vi "LiCor_poller.vi"(11 "LiCor session in":T1={"VISA resource out"="COM12", "error out"={"status"=FALSE, "code"=0, "source"=""}}) -> (0 "pCO2 out":dbl, 1 "data array":dbl[](array[numeric]), 2 "read string":string, 3 "LiCor session out":T1={"VISA resource out"="COM12", "error out"={"status"=FALSE, "code"=0, "source"=""}}, 4 "Integral out":dbl, 5 "actual bytes read":u32)   [LabVIEW 2010]
panel:
  # "LiCor Poller\n\nThis VI is a simple VI which completes a single poll of data from the LI-7000 LiCor instrument. It should follow a LiCor_init VI in whatever custom VI it is placed in - this will correctly initialize all the necessary values for successful operation. This VI spits out both raw data text as well as data in the form of an array."
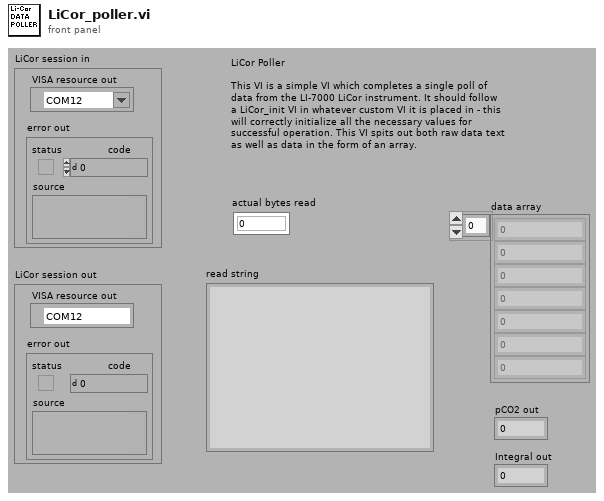
[diagram p1: front panel]
types:
  T1 = cluster{"VISA resource out":refnum<visa-resource-name>, "error out":errorcluster}
  T2 = cluster{"VISA session out":refnum<visa-resource-name>, "error out":errorcluster}
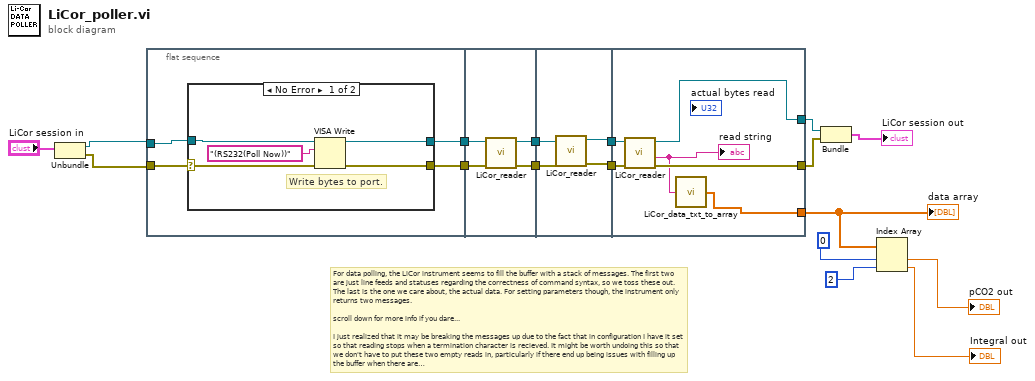
[diagram p0: block diagram]
diagram:
  # "For data polling, the LiCor instrument seems to fill the buffer with a stack of messages. The first two are just line feeds and statuses regarding the correctness of command syntax, so we toss these out. The last is the one we care about, the actual data. For setting parameters though, the instrument only returns two messages.\n\nscroll down for more info if you dare... \n\nI just realized that it may be breaking the messages up due to the fact that in configuration I have it set so that reading stops when a termination character is recieved. It might be worth undoing this so that we don't have to put these two empty reads in, particularly if there end up being issues with filling up the buffer when there are\n\nSorry for posting this as flow of thought, but if anyone is digging down this deep it may be useful. I just went into Advanced serial Write and Read and played around with some of the settings (ASRL End In, Supress End Enable, TermChar Enable and possible one or two others). Through some combination (which I think may have been accidental and I have not been able to reproduce though I haven't tried very hard - there may have been another setting I played with as well) I was able to get it to return both of the messages together (from a (Display(BackLt 1)) command), but I also got a timeout error from this. Trying to reset these values to ones that would make shut off the read termination, I was unable to reproduce the error, or get the read termination to end. Anyway, this isn't that important - I have things working. I just mention this in case someone has troubles down the road and needs to shoot them. It's also something of a matter of simple curiosity regarding what was causing the issues before. Nuff said..."
  n1 = Unbundle("LiCor session in") -> ("VISA resource out"=w10:refnum<visa-resource-name>, "error out"=w9:errorcluster)
  n2 = flat-sequence {
    tunnel: w10 -> [w21]
    tunnel: w9 -> [w20]
    tunnel: [w19] -> w17
    tunnel: [w18] -> w16
    tunnel: w17 -> [w32]
    tunnel: w16 -> [w31]
    tunnel: [w30] -> w15
    tunnel: [w29] -> w13
    tunnel: w15 -> [w36]
    tunnel: [w34] -> w14
    tunnel: w13 -> [w35]
    tunnel: [w33] -> w12
    tunnel: w14 -> [w42]
    tunnel: w12 -> [w41]
    tunnel: [w40] -> w8
    tunnel: [w39] -> w7
    tunnel: [w37] -> w3
    frame #0 {
      n3 = case shown="No Error" w20 {
        selector: w20 -> [w22 w28]
        tunnel: [w26 w27] -> w19
        tunnel: [w25 w28] -> w18
        tunnel: w21 -> [w23 w27]
        frame No Error {
          # "Write bytes to port."
          n4 = VISA Write(VISA resource name=w23, write buffer="(RS232(Poll Now))" ("string to write"), error in (no error)=w22) -> (VISA resource name out=w26:refnum<visa-resource-name>, error out=w25:errorcluster)  [unwired: 1 out]
        }
        frame Error {
        }
      }
    }
    frame #1 {
      n5 = call "LiCor_reader.vi"("error in"=w31, "VISA session in"=w32) -> ("error out"=w29:errorcluster, "VISA session out"=w30:refnum<visa-resource-name>)  [unwired: 6 in, 2 out]
    }
    frame #2 {
      n6 = call "LiCor_reader.vi"("error in"=w35, "VISA session in"=w36) -> ("error out"=w33:errorcluster, "VISA session out"=w34:refnum<visa-resource-name>)  [unwired: 6 in, 2 out]
    }
    frame #3 {
      n7 = call "LiCor_reader.vi"("error in"=w41, "VISA session in"=w42) -> ("error out"=w39:errorcluster, "read string"=w38:string, "VISA session out"=w40:refnum<visa-resource-name>)  [unwired: 6 in, 1 out]
      "read string" <- w38
      n8 = call "LiCor_data_txt_to_array.vi"("LiCor data string"=w38) -> ("Array"=w37:dbl[])
    }
  }
  n9 = Bundle("VISA session out"=w8, "error out"=w7) -> (→"LiCor session out":T2)  [unwired: 1 in]
  n10 = Index Array(array=w3, index #1=0, index #2=2) -> (element #1=→"pCO2 out":dbl, element #2=→"Integral out":dbl)
  "data array" <- w3
